vi "Spawn Primary Weapon.vi"(11 "Chmmr in":refnum<class "Chmmr.lvclass">) -> (2 "New Elements":refnum<class "Element.lvclass">[](array[class]), 3 "Chmmr out":refnum<class "Chmmr.lvclass">)   [LabVIEW 2021, in "Chmmr.lvclass"]
uses:
  Chmmr.lvclass
  C:/dev/LabVIEW/LabMelee/Source/Application Specific/Element/Element.lvclass
  Element/Element.lvclass
  Element/Element.lvclass/Element.ctl
  Motion/Motion.lvclass/Motion.ctl
  Chmmr.lvclass/Chmmr.ctl
  Vector 2D/Vector 2D.lvclass/Vector 2D.ctl
  Weapons/Laser/Laser.lvclass
  Actors/Main Controller/Actor/Player.ctl
  Actors/Main Controller/Actor/Main Controller Actor.lvclass
  Motion/Motion.lvclass
  Vector 2D/Vector 2D.lvclass
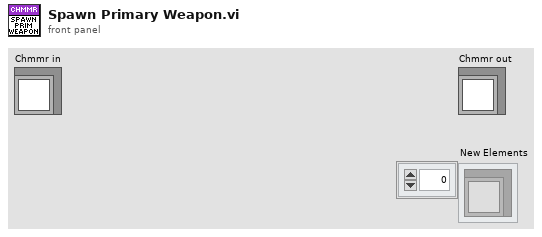
[diagram p1: front panel]
types:
  T1 = typedef "Main Controller Actor.lvclass/Player.ctl" = enum16{"1", "2"}
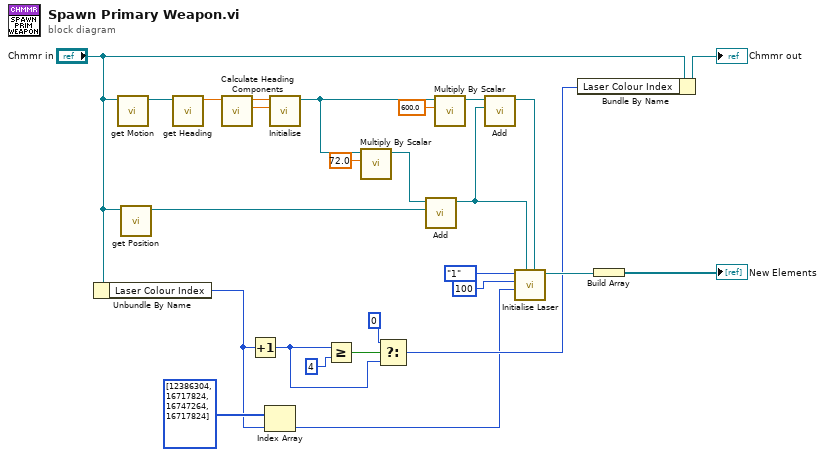
[diagram p0: block diagram]
diagram:
  n1 = Unbundle By Name("Chmmr in") -> ("Laser Colour Index"=w7:i32)
  n2 = call "get Motion.vi"("Element in"="Chmmr in") -> ("Motion"=w23:refnum<class "Motion.lvclass">)  [unwired: 10 in]
  n3 = call "get Position.vi"("Element in"="Chmmr in") -> ("Position"=w13:refnum<class "Vector 2D.lvclass">)  [unwired: 10 in]
  n4 = call "get Heading.vi"("Motion in"=w23) -> ("Heading [deg]"=w22:sgl)  [unwired: 10 in]
  n5 = call "Calculate Heading Components.vi"("Heading In [deg]"=w22) -> ("Sin Heading"=w20:sgl, "Cos Heading"=w21:sgl)  [unwired: 9 in]
  n6 = Increment(x=w7) -> (x+1=w4:i32)
  n7 = Index Array(array=u32[] [12386304, 16717824, 16747264, 16717824], index=w7) -> (element=w1:u32)
  n8 = call "Initialise.vi"("y"=w20, "x"=w21) -> ("Vector 2D out"=w14:refnum<class "Vector 2D.lvclass">)  [unwired: 9 in]
  n9 = Greater Or Equal?(x=w4, y=4) -> (x >= y?=w5:bool)
  n10 = call "Multiply By Scalar.vi"("x"=sgl 72.0, "A"=w14) -> ("Ax"=w12:refnum<class "Vector 2D.lvclass">)  [unwired: 9 in]
  n11 = Select(t=0 ("y"), s=w5, f=w4) -> (s? t:f=w2:i32)
  n12 = call "Add.vi"("B"=w13, "A"=w12) -> ("A+B"=w11:refnum<class "Vector 2D.lvclass">)  [unwired: 9 in]
  n13 = call "Multiply By Scalar.vi"("x"=sgl 600.0, "A"=w14) -> ("Ax"=w17:refnum<class "Vector 2D.lvclass">)  [unwired: 9 in]
  n14 = call "Add.vi"("B"=w11, "A"=w17) -> ("A+B"=w16:refnum<class "Vector 2D.lvclass">)  [unwired: 9 in]
  n15 = call "Initialise Laser.vi"("Endpoint"=w16, "Origin"=w11, "Colour"=w1, "Damage"=100, "Player"=Player."1") -> ("Laser out"=w26:refnum<class "Laser.lvclass">)  [unwired: 5 in, 1 out]
  n16 = Bundle By Name(cluster="Chmmr in", "Laser Colour Index"=w2) -> (→"Chmmr out":refnum<class "Chmmr.lvclass">)
  n17 = Build Array(w26) -> (→"New Elements":refnum<class "Laser.lvclass">[])
